vi "FTW-Menu-TagEncode.vi"(2 "Payload":string, 3 "Command":string, 4 "Class":string) -> (0 "Tag":string)   [LabVIEW 2014]
panel:
  # "Inputs"
  # "Outputs"
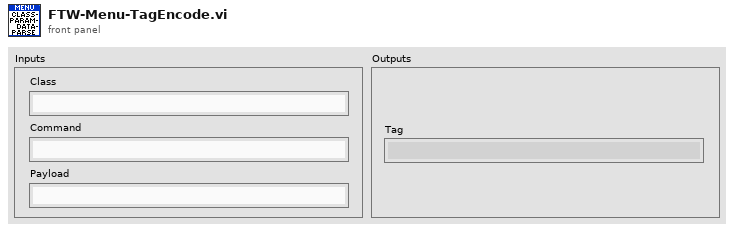
[diagram p1: front panel]
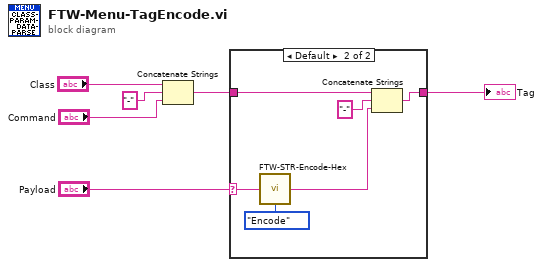
[diagram p0: block diagram]
diagram:
  n1 = Concatenate Strings("Class", "-" ("string"), "Command") -> (w2:string)
  n2 = case shown="Default" "Payload" {
    selector: "Payload" -> [_ w12]
    tunnel: w2 -> [w7 w10]
    tunnel: [w7 w11] -> w1
    frame "" {
    }
    frame Default {
      n3 = call "FTW-STR-Encode-Hex.vi"("Input"=w12, "Direction"=enum16{"Encode", "Decode"}."Encode") -> ("Output"=w9:string)
      n4 = Concatenate Strings(w10, "-" ("string"), w9) -> (w11:string)
    }
  }
  "Tag" <- w1
